vi "MES Server Check.vi"(8 "error in (no error)":errorcluster, 10 "MES Server":T1 items=["MES", "PD2", "PD3", "QA"], 11 "Local URL In":string) -> (0 "error out":errorcluster, 2 "Active?":bool, 3 "Url Tested Out":string)   [LabVIEW 2024]
uses:
  MES Servers.ctl
  C:/Users/bjames/Documents/GitHub/DataLogger/SubVIs/NetCheck.dll
  DataLogger/SubVIs/NetCheck.dll
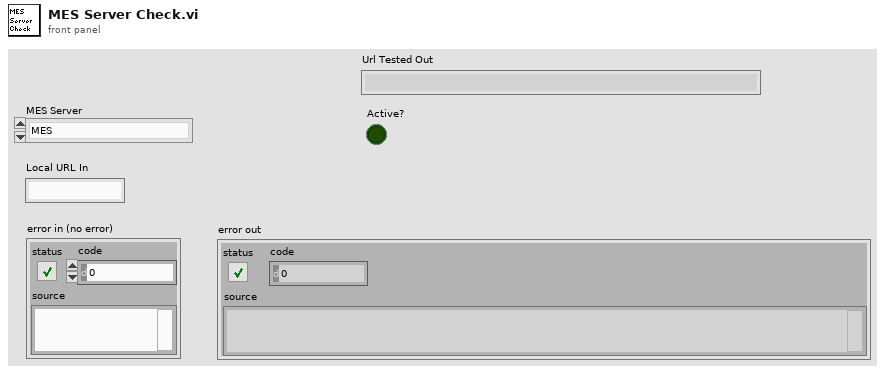
[diagram p1: front panel]
types:
  T1 = typedef "MES Servers.ctl" = u16
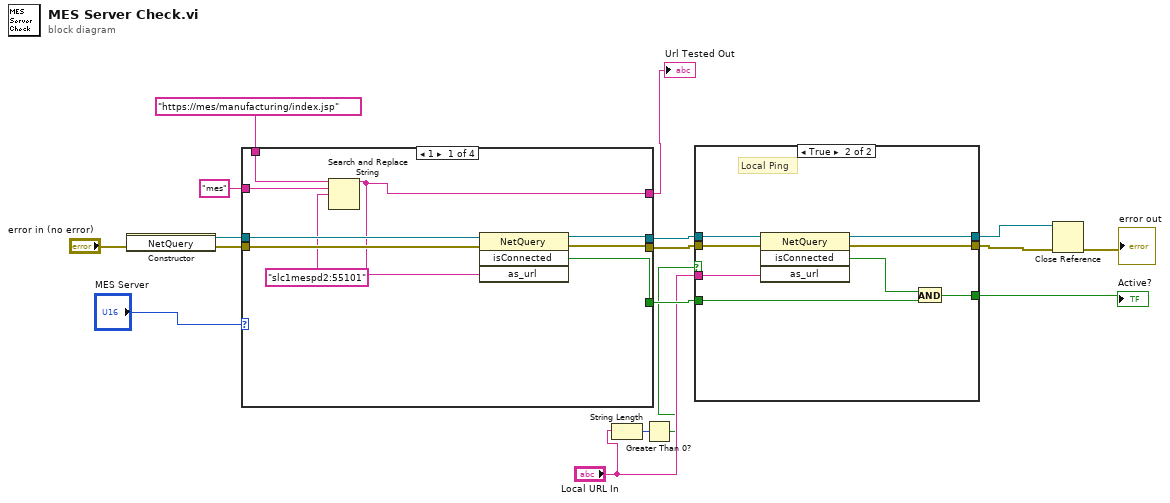
[diagram p0: block diagram]
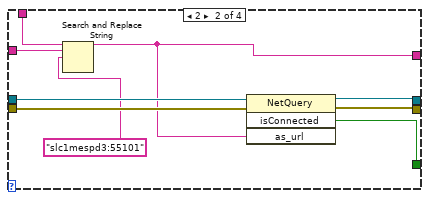
[diagram p3: hidden frame]
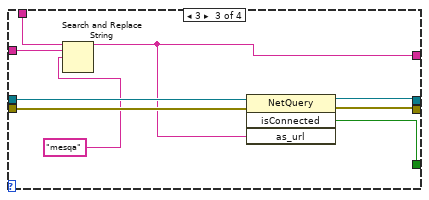
[diagram p4: hidden frame]
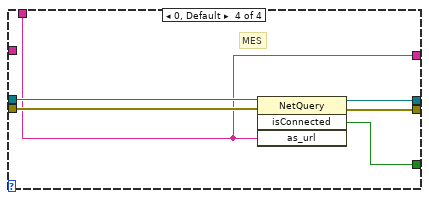
[diagram p5: hidden frame]
diagram:
  n1 = constructor class="NetQuery"(error in="error in (no error)") -> (reference out=w16:refnum<k24>, error out=w15:errorcluster)  [unwired: 2 in, 1 out]
  n2 = case shown="1" "MES Server" {
    tunnel: w16 -> [w26 w35 w44 w50]
    tunnel: w15 -> [w25 w34 w43 w49]
    tunnel: [w22 w31 w40 w48] -> w8
    tunnel: [w24 w33 w42 w47] -> w10
    tunnel: [w23 w32 w41 w46] -> w9
    tunnel: [w18 w27 w36 w45] -> w4
    tunnel: "https://mes/manufacturing/index.jsp" -> [w21 w30 w39 w45]
    tunnel: "mes" -> [w20 w29 w38 _]
    frame 1 {
      n3 = Search and Replace String(input string=w21, search string=w20, replace string="slc1mespd2:55101") -> (result string=w18:string)  [unwired: 5 in, 3 out]
      n4 = invoke class="NetQuery" method="isConnected"(reference=w26, error in=w25, "as_url"=w18) -> (reference out=w24:refnum<k24>, error out=w23:errorcluster, "isConnected"=w22:bool)  [unwired: 1 in, 1 out]
    }
    frame 2 {
      n5 = Search and Replace String(input string=w30, search string=w29, replace string="slc1mespd3:55101") -> (result string=w27:string)  [unwired: 5 in, 3 out]
      n6 = invoke class="NetQuery" method="isConnected"(reference=w35, error in=w34, "as_url"=w27) -> (reference out=w33:refnum<k24>, error out=w32:errorcluster, "isConnected"=w31:bool)  [unwired: 1 in, 1 out]
    }
    frame 3 {
      n7 = Search and Replace String(input string=w39, search string=w38, replace string="mesqa") -> (result string=w36:string)  [unwired: 5 in, 3 out]
      n8 = invoke class="NetQuery" method="isConnected"(reference=w44, error in=w43, "as_url"=w36) -> (reference out=w42:refnum<k24>, error out=w41:errorcluster, "isConnected"=w40:bool)  [unwired: 1 in, 1 out]
    }
    frame 0, Default {
      # "MES"
      n9 = invoke class="NetQuery" method="isConnected"(reference=w50, error in=w49, "as_url"=w45) -> (reference out=w47:refnum<k24>, error out=w46:errorcluster, "isConnected"=w48:bool)  [unwired: 1 in, 1 out]
    }
  }
  "Url Tested Out" <- w4
  n10 = String Length(string="Local URL In") -> (length=w3:i32)
  n11 = Greater Than 0?(x=w3) -> (x > 0?=w1:bool)
  n12 = case shown="True" w1 {
    tunnel: w10 -> [w53 w61]
    tunnel: w9 -> [w52 w60]
    tunnel: w8 -> [w51 w59]
    tunnel: [w51 w58] -> w7
    tunnel: [w52 w57] -> w6
    tunnel: [w53 w56] -> w5
    tunnel: "Local URL In" -> [_ w55]
    frame False {
    }
    frame True {
      # "Local Ping"
      n13 = invoke class="NetQuery" method="isConnected"(reference=w61, error in=w60, "as_url"=w55) -> (reference out=w56:refnum<k24>, error out=w57:errorcluster, "isConnected"=w54:bool)  [unwired: 1 in, 1 out]
      n14 = And(x=w54, y=w59) -> (x .and. y?=w58:bool)
    }
  }
  "Active?" <- w7
  n15 = Close Reference(reference=w5, error in (no error)=w6) -> (error out=→"error out":errorcluster)
